vi "convertToKeyValuePair_double.vi"(8 "error in (no error)":errorcluster, 9 "precision (0)":u8, 10 "value":dbl, 11 "name":string) -> (0 "error out":errorcluster, 3 "string converted":string)   [LabVIEW 2018]
doc: "Convert a double numeric into a key value pair as string."
uses:
  convertToKeyValuePair_string.vi
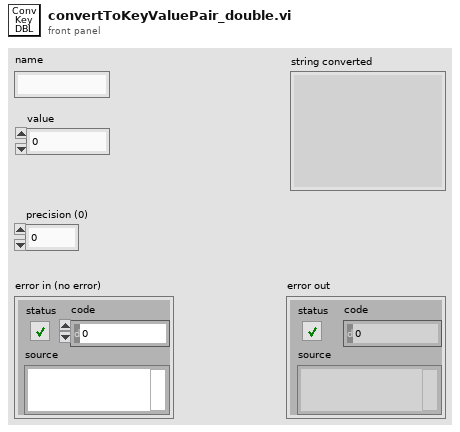
[diagram p1: front panel]
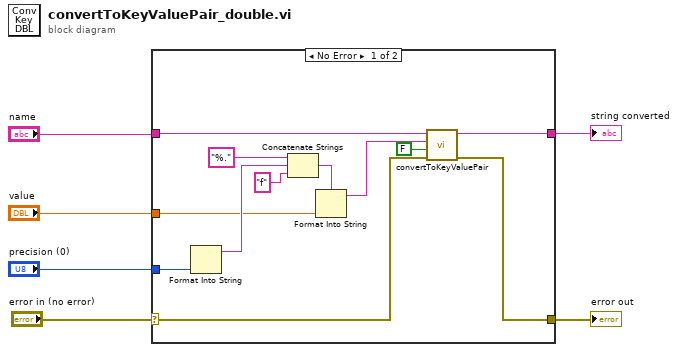
[diagram p0: block diagram]
diagram:
  n1 = case shown="No Error" "error in (no error)" {
    selector: "error in (no error)" -> [w9 w19]
    tunnel: [w12 _] -> w6
    tunnel: "name" -> [w10 _]
    tunnel: "precision (0)" -> [w18 _]
    tunnel: [w8 w19] -> w2
    tunnel: "value" -> [w13 _]
    frame No Error {
      n2 = Format Into String(w18) -> (resulting string=w15:string)  [unwired: 3 in, 1 out]
      n3 = Concatenate Strings("%." ("format string"), w15, "f" ("format string")) -> (w14:string)
      n4 = Format Into String(format string=w14, w13) -> (resulting string=w11:string)  [unwired: 2 in, 1 out]
      n5 = call-poly "convertToKeyValuePair.vi"("error in (no error)"=w9, "double quotes (T)"=FALSE, "value"=w11, "name"=w10) -> ("error out"=w8:errorcluster, "string converted"=w12:string)  [unwired: 6 in]
    }
    frame Error {
    }
  }
  "error out" <- w2
  "string converted" <- w6
